vi "PrepLineObjectArray_write_and_unlock_queue.vi"(8 "error in (no error)":errorcluster, 11 "PrepLineObjArray":refnum<class "PrepLineObject.lvclass">[](array[class])) -> (0 "error out":errorcluster)   [LabVIEW 2018]
doc: "The VI wites the PrepLineObject Array into the named queue, that stores the array. By writing the data into the queue, the array/queue is ready to be accessed by another process"
uses:
  Classes/PrepLineObject/PrepLineObject.lvclass
  global variables.vi
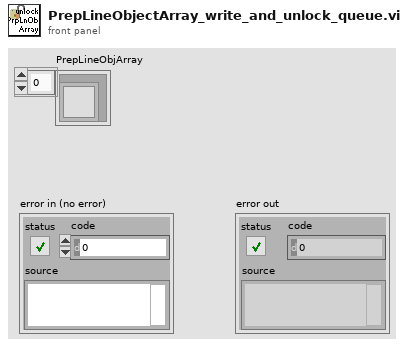
[diagram p1: front panel]
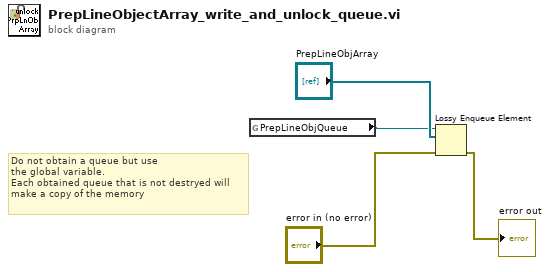
[diagram p0: block diagram]
diagram:
  # "Do not obtain a queue but use\nthe global variable.\nEach obtained queue that is not destryed will\nmake a copy of the memory"
  n1 = global read "global variables.vi" "PrepLineObjQueue"() -> (w2:refnum<queue>)
  n2 = Lossy Enqueue Element(queue=w2, element="PrepLineObjArray", error in (no error)="error in (no error)") -> (error out=→"error out":errorcluster)  [unwired: 3 out]
